vi "User Log Write.vi"(8 "Error Into File Write":errorcluster, 9 "User Info to Write":string, 11 "File Location of User Logs":path) -> (0 "File Write Error Out":errorcluster)   [LabVIEW 2020]
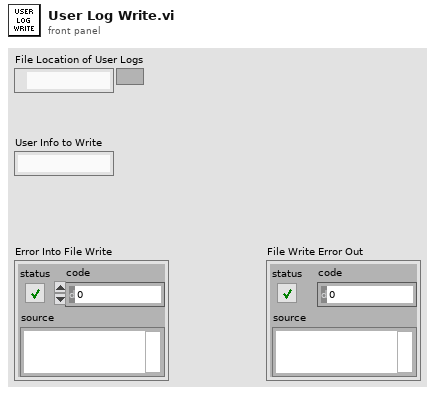
[diagram p1: front panel]
types:
  T1 = enum16{"open", "replace", "create", "open or create", "replace or create", "replace or create with confirmation"}
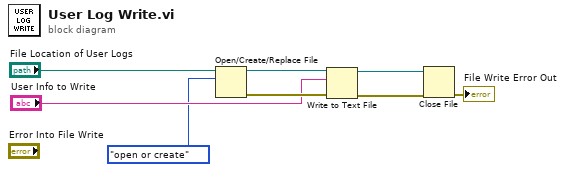
[diagram p0: block diagram]
diagram:
  n1 = Open/Create/Replace File(file path (use dialog)="File Location of User Logs", operation (0:open)=T1."open or create") -> (refnum out=w6:refnum<file>, error out=w4:errorcluster)  [unwired: 4 in, 1 out]
  n2 = Write to Text File(file (use dialog)=w6, text="User Info to Write", error in=w4) -> (refnum out=w5:refnum<file>, error out=w8:errorcluster)  [unwired: 1 in, 1 out]
  n3 = Close File(refnum=w5, error in=w8) -> (error out=→"File Write Error Out":errorcluster)  [unwired: 1 out]
